vi "Self Configure.vi"(8 "error in":errorcluster, 11 "Multimeter in":refnum<class "Multimeter.lvclass">) -> (0 "error out":errorcluster, 3 "Multimeter out":refnum<class "Multimeter.lvclass">)   [LabVIEW 2019, in "Multimeter.lvlib" / "Multimeter.lvclass"]
doc: "Children of Instruments must override this routine and call the parent method. \nThis routine is implemented to allow each instrument to read its specific configuration keys and implement any default configuration settings.\n\nThis routine already calls Connect and Self Test Routines."
uses:
  Library/Multimeter.lvclass
  builds/Instruments/Instruments.lvlibp/Library/Instruments.lvclass
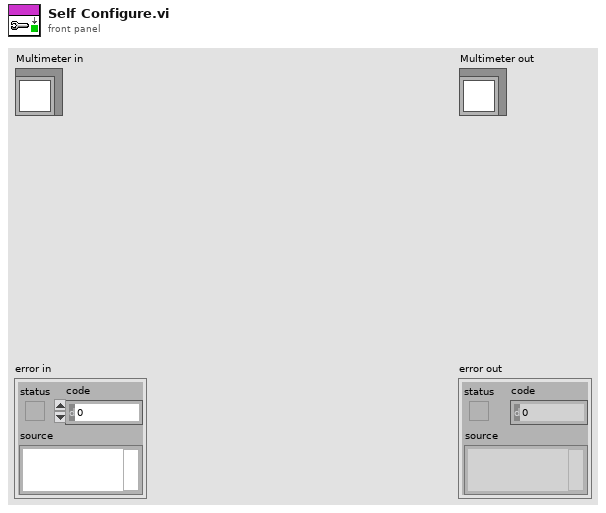
[diagram p1: front panel]
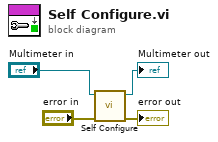
[diagram p0: block diagram]
diagram:
  n1 = call-parent "Self Configure.vi"("error in"="error in", "Instruments in"="Multimeter in") -> ("error out"=→"error out":errorcluster, "Instruments out"=→"Multimeter out":refnum<class "Multimeter.lvclass">)  [unwired: 8 in]
